vi "calibrationElectrometer_getEvent_settingVersions.vi"(8 "error in (no error)":errorcluster, 11 "logevent_settingVersions_Ctl":T1={"timestamp"=0.0, "recommendedSettingsVersion"="                                                                                                                                                                                                                                                                ", "recommendedSettingLabels"="", "priority"=0}) -> (0 "error out":errorcluster, 2 "function return":i32, 3 "logevent_settingVersions_Ctl out":T1={"timestamp"=0.0, "recommendedSettingsVersion"="                                                                                                                                                                                                                                                                ", "recommendedSettingLabels"="", "priority"=0})   [LabVIEW 2016, in "SALLV_calibrationElectrometer.lvlib"]
doc: "int calibrationElectrometer_shm_getEvent_settingVersionsLV(calibrationElectrometer_logevent_settingVersionsLV *logevent_settingVersions_Ctl );"
uses:
  SALLV_calibrationElectrometer.lvlib
  DataTypes/logevent_settingVersions.ctl
  SALLV_calibrationElectrometer.so
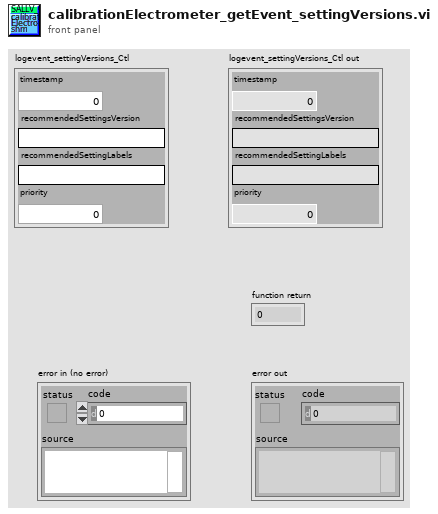
[diagram p1: front panel]
types:
  T1 = typedef "SALLV_calibrationElectrometer.lvlib/logevent_settingVersions.ctl" = cluster{"timestamp":dbl, "recommendedSettingsVersion":string, "recommendedSettingLabels":string, "priority":i32}
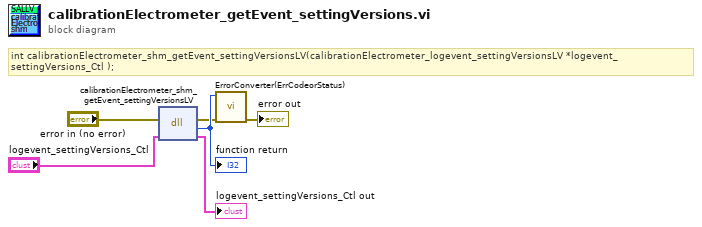
[diagram p0: block diagram]
diagram:
  # "int calibrationElectrometer_shm_getEvent_settingVersionsLV(calibrationElectrometer_logevent_settingVersionsLV *logevent_settingVersions_Ctl );"
  n1 = dll-call lib="home/andres/Desktop/SAL_calibrationElectrometer/SALLV_calibrationElectrometer.*" fn="calibrationElectrometer_shm_getEvent_settingVersionsLV"(error in="error in (no error)", "logevent_settingVersions_Ctl"="logevent_settingVersions_Ctl") -> (error out=w2:errorcluster, w6:i32, "logevent_settingVersions_Ctl"=→"logevent_settingVersions_Ctl out":T1)  [unwired: 2 in, 1 out]
  "function return" <- w6
  n2 = call "ErrorConverter(ErrCodeorStatus).vi"("error in (no error)"=w2, "error code"=w6) -> ("error out"=→"error out":errorcluster)  [unwired: 9 in]
